vi "Zip Array of Files.vi"(8 "error in (no error)":errorcluster, 10 "Target Zip Filename":path, 11 "Files to Zip":path[](array[path])) -> (0 "error out":errorcluster)   [LabVIEW 2013]
panel:
  # "1"
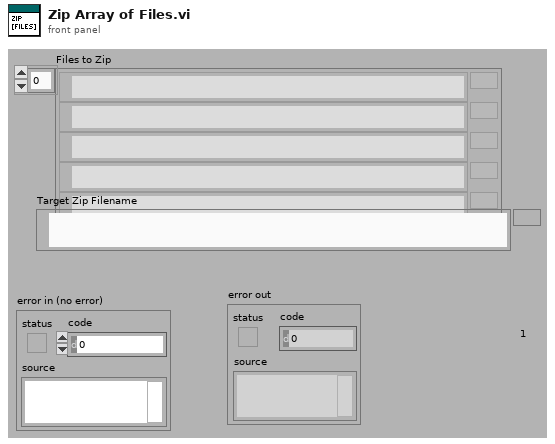
[diagram p1: front panel]
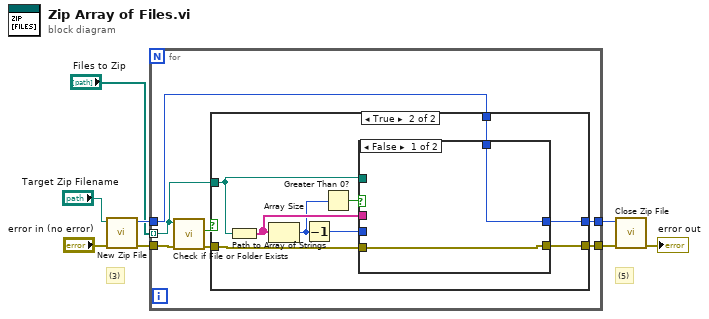
[diagram p0: block diagram]
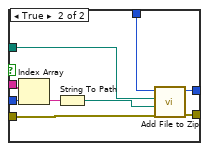
[diagram p3: hidden frame]
diagram:
  # "(5)"
  # "(3)"
  n1 = call <vilib>:"New Zip File.vi"("error in (no error)"="error in (no error)", "target"="Target Zip Filename") -> ("error out"=w7:errorcluster, "zip file out"=w8:i64)  [unwired: 1 in, 3 out]
  n2 = for {
    tunnel: "Files to Zip" -> [w10] mode=indexing
    tunnel: w8 -> [w15]
    tunnel: w7 -> [w12]
    tunnel: [w14] -> w6
    tunnel: [w13] -> w5
    n3 = call <vilib>:"Check if File or Folder Exists.vi"("error in (no error)"=w12, "path"=w10) -> ("error out"=w11:errorcluster, "file or folder exists?"=w9:bool)  [unwired: 7 in, 1 out]
    n4 = case shown="True" w9 {
      tunnel: w15 -> [w16 w26]
      tunnel: [w17 w25] -> w14
      tunnel: [w16 w24] -> w13
      tunnel: w11 -> [w17 w21]
      tunnel: w10 -> [_ w20]
      frame False {
      }
      frame True {
        n5 = Path to Array of Strings(0:w20) -> (2:w23:string[])  [unwired: 1 out]
        n6 = Array Size(array=w23) -> (size(s)=w18:i32)
        n7 = Decrement(x=w18) -> (x-1=w22:i32)
        n8 = Greater Than 0?(x=w18) -> (x > 0?=w19:bool)
        n9 = case shown="False" w19 {
          tunnel: w26 -> [w28 w37]
          tunnel: [w27 w36] -> w25
          tunnel: [w28 w35] -> w24
          tunnel: w23 -> [_ w34]
          tunnel: w22 -> [_ w31]
          tunnel: w21 -> [w27 w30]
          tunnel: w20 -> [_ w29]
          frame False {
          }
          frame True {
            n10 = Index Array(array=w34, index=w31) -> (element=w33:string)
            n11 = String To Path(string=w33) -> (path=w32:path)
            n12 = call <vilib>:"Add File to Zip.vi"("error in (no error)"=w30, "destination path in zip"=w32, "source file path"=w29, "zip file in"=w37) -> ("error out"=w36:errorcluster, "zip file out"=w35:i64)  [unwired: 6 out]
          }
        }
      }
    }
  }
  n13 = call <vilib>:"Close Zip File.vi"("error in (no error)"=w6, "zip file in"=w5) -> ("error out"=→"error out":errorcluster)  [unwired: 1 in, 4 out]
